vi "TeachableMachineHtmlCreate.vi"() -> ()   [LabVIEW 2021]
uses:
  <vilib>/Utility/NIReport.llb/Report Type.ctl
  <vilib>/Platform/browser.llb/Open URL in Default Browser (string).vi
  <vilib>/Utility/NIReport.llb/NI_report.lvclass
  <vilib>/Utility/NIReport.llb/NI_ReportGenerationCore.lvlib
panel:
  out "error IO":errorcluster
  out "connection ID":refnum<k5>
  out "data out":string
  in  "stop":bool
  out "URL out":string
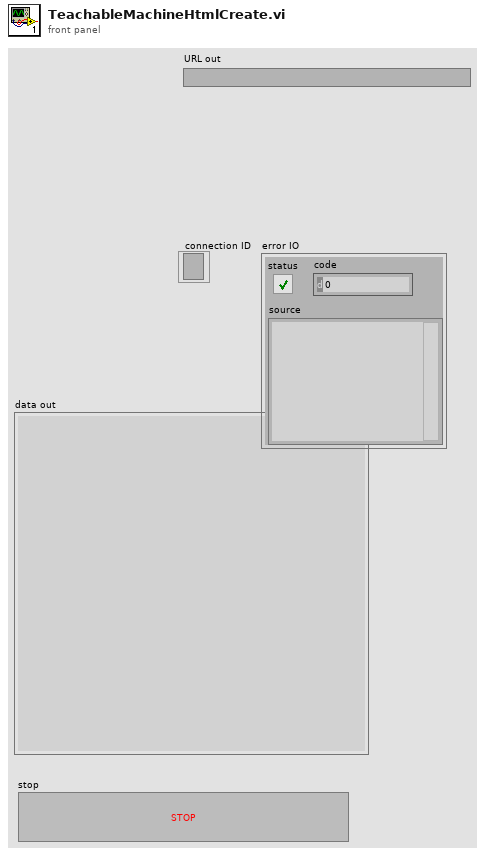
[diagram p1: front panel]
types:
  T1 = typedef "NI_ReportGenerationCore.lvlib/Report Type.ctl" = enum16{"HTML", "Word", "Excel"}
  T2 = enum16{"Standard", "Buffered", "CRLF", "Immediate"}
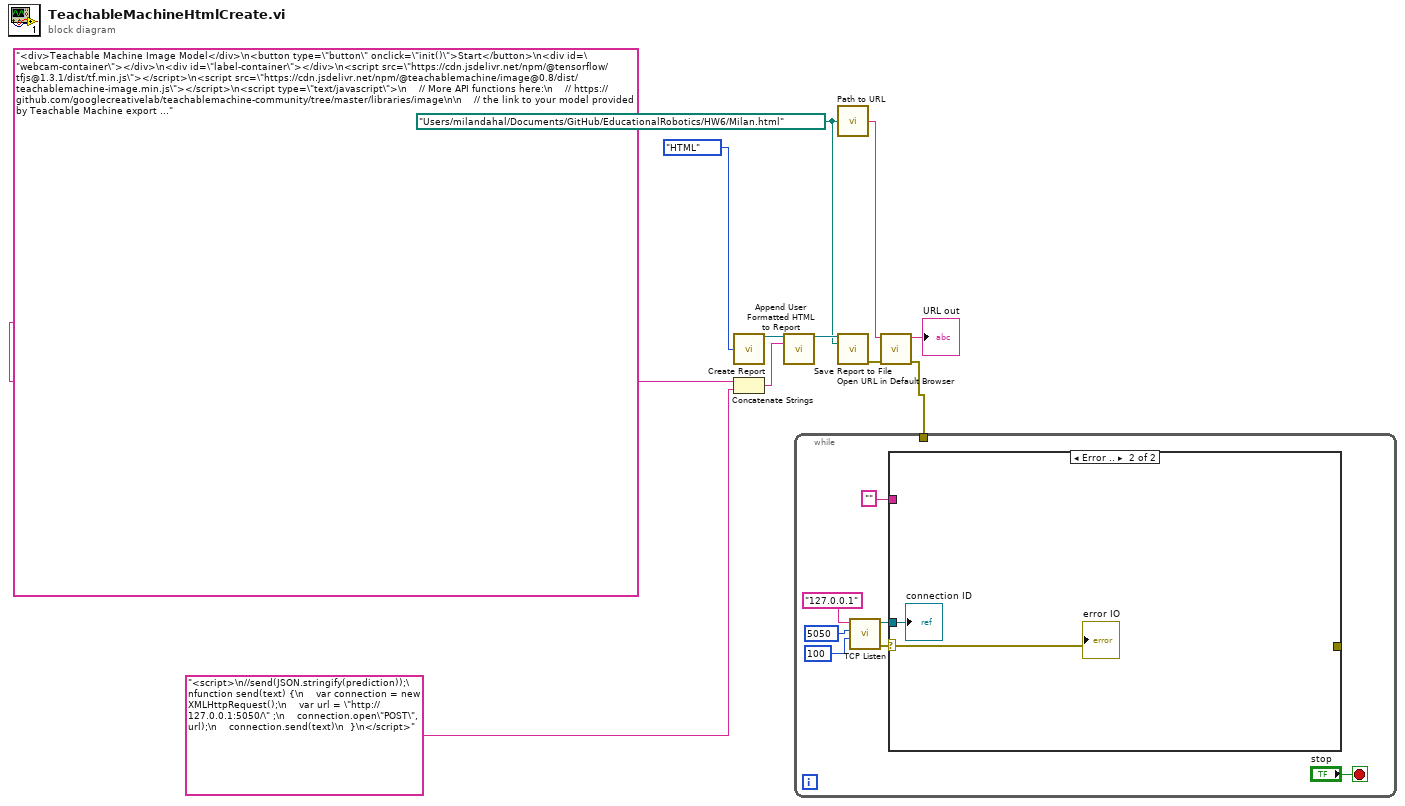
[diagram p0: block diagram]
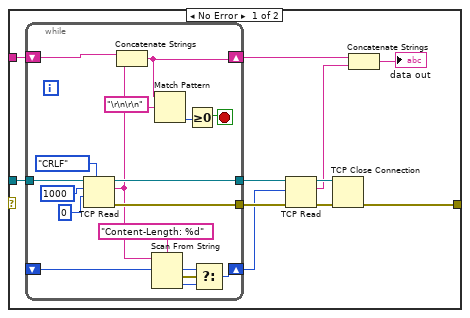
[diagram p2: hidden frame]
diagram:
  w6 = path "/Users/milandahal/Documents/GitHub/EducationalRobotics/HW6/Milan.html" ("report file path")
  n1 = call <vilib>:"Create Report.vi"("Report Type"=Report_Type."HTML") -> ("report out"=w10:refnum<class "NI_report.lvclass">)  [unwired: 13 in, 1 out]
  n2 = Concatenate Strings("<div>Teachable Machine Image Model</div>\n<button type=\"button\" onclick=\"init()\">Start</button>\n<div id=\"webcam-container\"></div>\n<div id=\"label-container\"></div>\n<script src=\"https://cdn.jsdelivr.net/npm/@tensorflow/tfjs@1.3.1/dist/tf.min.js\"></script>\n<script src=\"https://cdn.jsdelivr.net/npm/@teachablemachine/image@0.8/dist/teachablemachine-image.min.js\"></script>\n<script type=\"text/javascript\">\n    // More API functions here:\n    // https://github.com/googlecreativelab/teachablemachine-community/tree/master/libraries/image\n\n    // the link to your model provided by Teachable Machine export panel\n    const URL = \"https://teachablemachine.withgoogle.com/models/9m5FPP7a0/\";\n\n    let model, webcam, labelContainer, maxPredictions;\n\n    // Load the image model and setup the webcam\n    async function init() {\n        const modelURL = URL + \"model.json\";\n        const metadataURL = URL + \"metadata.json\";\n\n        // load the model and metadata\n        // Refer to tmImage.loadFromFiles() in the API to support files from a file picker\n        // or files from your local hard drive\n        // Note: the pose library adds \"tmImage\" object to your window (window.tmImage)\n        model = await tmImage.load(modelURL, metadataURL);\n        maxPredictions = model.getTotalClasses();\n\n        // Convenience function to setup a webcam\n        const flip = true; // whether to flip the webcam\n        webcam = new tmImage.Webcam(200, 200, flip); // width, height, flip\n        await webcam.setup(); // request access to the webcam\n        await webcam.play();\n        window.requestAnimationFrame(loop);\n\n        // append elements to the DOM\n        document.getElementById(\"webcam-container\").appendChild(webcam.canvas);\n        labelContainer = document.getElementById(\"label-container\");\n        for (let i = 0; i < maxPredictions; i++) { // and class labels\n            labelContainer.appendChild(document.createElement(\"div\"));\n        }\n    }\n\n    async function loop() {\n        webcam.update(); // update the webcam frame\n        await predict();\n        window.requestAnimationFrame(loop);\n    }\n\n    // run the webcam image through the image model\n    async function predict() {\n        // predict can take in an image, video or canvas html element\n        const prediction = await model.predict(webcam.canvas);\n        for (let i = 0; i < maxPredictions; i++) {\n            const classPrediction =\n                prediction[i].className + \": \" + prediction[i].probability.toFixed(2);\n            labelContainer.childNodes[i].innerHTML = classPrediction;\n        }\n\n    }\n\nsend(JSON.stringify(prediction));\n</script>\n" ("HTML text"), "<script>\n//send(JSON.stringify(prediction));\nfunction send(text) {\n    var connection = new XMLHttpRequest();\n    var url = \"http://127.0.0.1:5050/\" ;\n    connection.open\"POST\", url);\n    connection.send(text)\n  }\n</script>" ("string")) -> (w2:string)
  n3 = call-dynamic "Append User Formatted HTML to Report.vi"("report in"=w10, "HTML text"=w2) -> ("report out"=w7:refnum<class "NI_report.lvclass">)  [unwired: 12 in, 1 out]
  n4 = call <vilib>:"Path to URL.vi"("path"=w6) -> ("url"=w9:string)
  n5 = call-dynamic "Save Report to File.vi"("report in"=w7, "report file path"=w6) -> ("error out"=w8:errorcluster)  [unwired: 12 in, 1 out]
  n6 = call-poly <vilib>:"Open URL in Default Browser.vi"("error in (no error)"=w8, "URL"=w9) -> ("error out"=w1:errorcluster, "URL out"=→"URL out":string)  [unwired: 4 in]
  n7 = while {
    tunnel: w1 -> [_]
    stop <- "stop" stop-if-true
    n8 = call <vilib>:"TCP Listen.vi"("timeout ms (wait forever: -1)"=100, "port"=u16 5050, "service name"="127.0.0.1") -> ("error out"=w14:errorcluster, "connection ID"=w17:refnum<k5>)  [unwired: 4 in, 3 out]
    n9 = case shown="Error .." w14 {
      selector: w14 -> [_ w47]
      tunnel: w17 -> [w28 w48]
      tunnel: [w29 _] -> _
      tunnel: "" -> [w19 _]
      frame No Error {
        n10 = while {
          tunnel: [w43] -> w26
          tunnel: w28 -> [w44]
          tunnel: [w42] -> w27
          shift-right: [w36] -> w22
          shift-left: w19 -> [w41]
          shift-right: [w31] -> w23
          shift-left: _ -> [w32]
          stop <- w38 stop-if-true
          n11 = TCP Read(connection ID=w44, bytes to read=1000, 7:T2."CRLF" ("mode (standard)"), 9:0 ("timeout ms (25000)")) -> (connection ID out=w42:refnum<k5>, data out=w30:string, error out=w43:errorcluster)  [unwired: 1 in]
          n12 = Concatenate Strings(w41, w30) -> (w36:string)
          n13 = Scan From String(format string="Content-Length: %d", input string=w30) -> (error out=w34:errorcluster, output 1=w33:i32)  [unwired: 3 in, 2 out]
          n14 = Match Pattern(string=w36, regular expression="\r\n\r\n") -> (offset past match=w39:i32)  [unwired: 1 in, 3 out]
          n15 = Greater Or Equal To 0?(x=w39) -> (x >= 0?=w38:bool)
          n16 = Select(t=w32, s=w34, f=w33) -> (s? t:f=w31:i32)
        }
        n17 = TCP Read(connection ID=w27, bytes to read=w23, error in (no error)=w26) -> (connection ID out=w24:refnum<k5>, data out=w21:string, error out=w25:errorcluster)  [unwired: 2 in]
        n18 = TCP Close Connection(connection ID=w24, error in (no error)=w25) -> (error out=w29:errorcluster)  [unwired: 1 in, 1 out]
        n19 = Concatenate Strings(w22, w21) -> (→"data out":string)
      }
      frame Error {
        "connection ID" <- w48
        "error IO" <- w47
      }
    }
  }
